vi "Update Point Marker.vi"(8 "Error In":errorcluster, 11 "Route Index":i32) -> (0 "Error Out":errorcluster)   [LabVIEW 2014]
uses:
  C:/Robotic Systems/Products/Surveyor/Software/Ground Station/Data/Mapping DLL/GMap.NET.WindowsForms.dll
  Data/Mapping DLL/GMap.NET.WindowsForms.dll
  Reference/SubVI/GMap DLL Refernce.vi
  Reference/SubVI/Main Map Control Refernce.vi
  Missions/FGVs/Currently Selected Virtual WP/Methods/Get Current Virtual Waypoint.vi
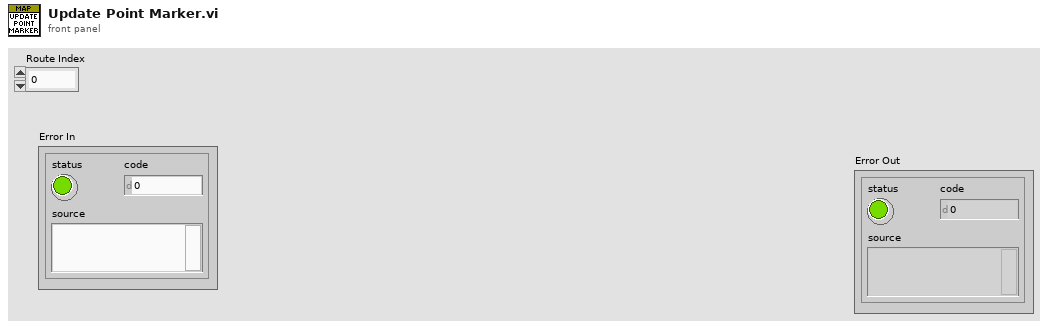
[diagram p1: front panel]
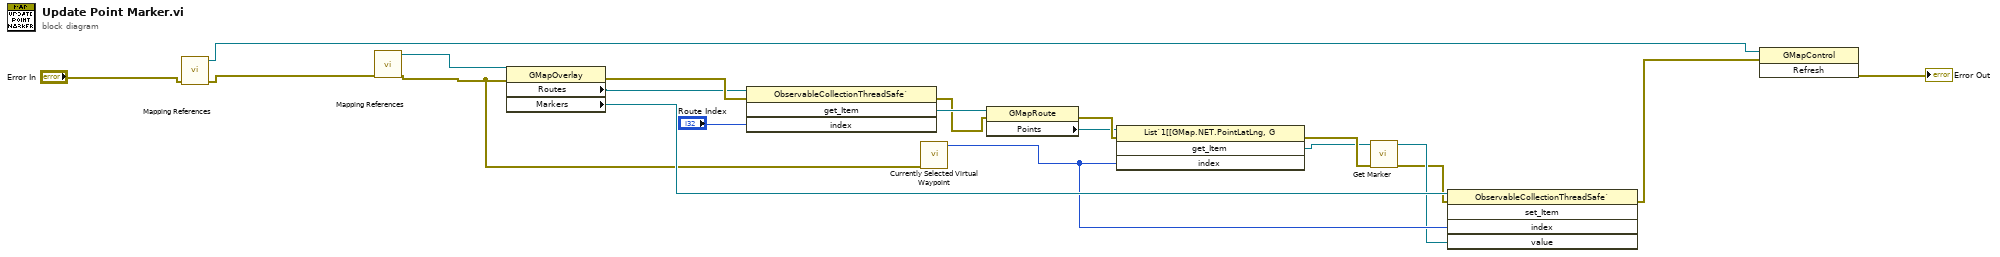
[diagram p0: block diagram]
diagram:
  n1 = call-poly "Mapping References.vi"("Error In"="Error In") -> ("Error Out"=w16:errorcluster, "GMap DLL Reference"=w14:refnum<k24>)  [unwired: 9 in]
  n2 = call-poly "Mapping References.vi"("Error In"=w16) -> ("Error Out"=w7:errorcluster, "Main Map Reference"=w17:refnum<k24>)  [unwired: 9 in]
  n3 = property class="GMapOverlay"(reference=w17, error in=w7) -> (error out=w20:errorcluster, "Routes"=w12:refnum<k24>, "Markers"=w11:refnum<k24>)  [unwired: 1 out]
  n4 = invoke class="ObservableCollectionThreadSafe`" method="get_Item"(reference=w12, error in=w20, "index"="Route Index") -> (error out=w10:errorcluster, "get_Item"=w19:refnum<k24>)  [unwired: 1 in, 2 out]
  n5 = call-poly "Currently Selected Virtual Waypoint.vi"("Error In"=w7) -> ("Waypoint Index Out"=w6:u32)  [unwired: 9 in, 1 out]
  n6 = property class="GMapRoute"(reference=w19, error in=w10) -> (error out=w9:errorcluster, "Points"=w8:refnum<k24>)  [unwired: 1 out]
  n7 = invoke class="List`1[[GMap.NET.PointLatLng, G" method="get_Item"(reference=w8, error in=w9, "index"=w6) -> (error out=w5:errorcluster, "get_Item"=w4:refnum<k24>)  [unwired: 1 in, 2 out]
  n8 = call "Get Marker.vi"("Error In"=w5, "Point"=w4) -> ("error out"=w2:errorcluster, "new reference"=w3:refnum<k24>)  [unwired: 8 in]
  n9 = invoke class="ObservableCollectionThreadSafe`" method="set_Item"(reference=w11, error in=w2, "index"=w6, "value"=w3) -> (error out=w1:errorcluster)  [unwired: 1 in, 4 out]
  n10 = invoke class="GMapControl" method="Refresh"(reference=w14, error in=w1) -> (error out=→"Error Out":errorcluster)  [unwired: 1 in, 2 out]
